vi "Temperature sub final.vi"(8 "error in (no error)":errorcluster, 10 "Numeric 3":i32, 11 "LINX Resource":T1) -> (2 "Numeric 2":i32, 3 "Numeric":dbl)   [LabVIEW 2020]
uses:
  <vilib>/MakerHub/LINX/Private/Type Defs/LINX Ref.ctl
  <vilib>/MakerHub/LINX/Private/Type Defs/Platform.ctl
  <vilib>/MakerHub/LINX/Private/Type Defs/Interface.ctl
  <vilib>/MakerHub/LINX/Private/Device/Type Defs/LINX Device Config.ctl
  <vilib>/MakerHub/LINX/Private/Device/Type Defs/TCP Config.ctl
  <vilib>/MakerHub/LINX/Private/Device/Type Defs/Channels.ctl
  <vilib>/MakerHub/LINX/Public/Peripherals/Analog/Analog Read 1 Chan.vi
  <vilib>/MakerHub/LINX/Public/Peripherals/Analog/Analog Read N Chans.vi
  <vilib>/MakerHub/LINX/Private/Local IO/LinxAnalogRead.vi
  <vilib>/MakerHub/LINX/Public/Utilities/Check Channel.vi
  <vilib>/MakerHub/LINX/Private/Utilties/Generate Error.vi
  <vilib>/MakerHub/LINX/LMH-LINX.lvlib
  <vilib>/MakerHub/LINX/Private/Device/Device.lvlib
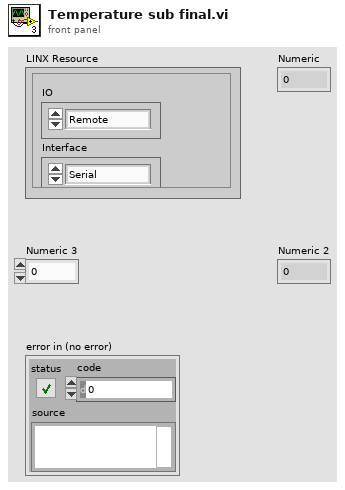
[diagram p1: front panel]
types:
  T1 = typedef "LMH-LINX.lvlib/LINX Ref.ctl" = cluster{"IO":T2, "Interface":T3, "LINX Device Config":T4}
  T2 = typedef "LMH-LINX.lvlib/Platform.ctl" = enum16{"Remote", "Local"}
  T3 = typedef "LMH-LINX.lvlib/Interface.ctl" = enum16{"Serial", "TCP"}
  T4 = typedef "LMH-LINX.lvlib/Device.lvlib/LINX Device Config.ctl" = cluster{"Interface":T3, "COM Port":refnum<visa-resource-name>, "TCP Configuration":T5, "Device Family":u8, "Device ID":u8, "Device Name":string, "TCP Ref":refnum<k5>, "Channels":T6}
  T5 = typedef "LMH-LINX.lvlib/Device.lvlib/TCP Config.ctl" = cluster{"IP Address":string, "Port":u16}
  T6 = typedef "LMH-LINX.lvlib/Channels.ctl" = cluster{"DI":u8[], "DO":u8[], "AI":u8[], "AO":u8[], "PWM":u8[], "QE":u8[], "UART":u8[], "I2C 2":u8[], "SPI":u8[], "CAN":u8[], "Servo":u8[], "AI Ref (V)":dbl, "AI Resolution (Bits)":u8, "AO Ref (V)":dbl, "AO Resolution (Bits)":u8}
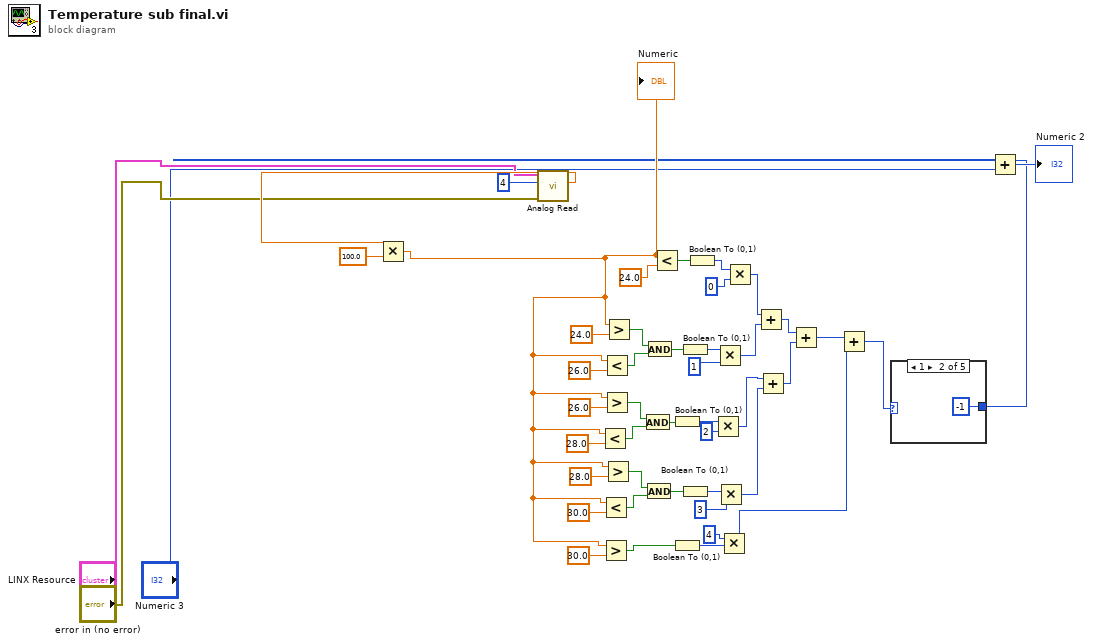
[diagram p0: block diagram]
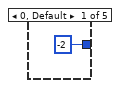
[diagram p2: hidden frame]
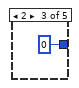
[diagram p3: hidden frame]
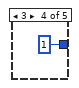
[diagram p4: hidden frame]
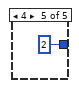
[diagram p5: hidden frame]
diagram:
  n1 = call-poly <vilib>:"Analog Read.vi"("Error In"="error in (no error)", "Analog Channel"=u8 4, "LINX Resource"="LINX Resource") -> ("Voltage"=w47:dbl)  [unwired: 5 in, 3 out]
  n2 = Multiply(x=w47, y=100.0) -> (x*y=w6:dbl)
  "Numeric" <- w6
  n3 = Less?(x=w6, y=28.0) -> (x < y?=w15:bool)
  n4 = Less?(x=w6, y=30.0) -> (x < y?=w19:bool)
  n5 = Greater?(x=w6, y=30.0) -> (0:w23:bool)
  n6 = Less?(x=w6, y=26.0) -> (x < y?=w11:bool)
  n7 = Greater?(x=w6, y=26.0) -> (0:w16:bool)
  n8 = Greater?(x=w6, y=28.0) -> (0:w20:bool)
  n9 = Greater?(x=w6, y=24.0) -> (0:w12:bool)
  n10 = And(x=w16, y=w15) -> (x .and. y?=w25:bool)
  n11 = And(x=w20, y=w19) -> (x .and. y?=w24:bool)
  n12 = And(x=w12, y=w11) -> (x .and. y?=w26:bool)
  n13 = Less?(x=w6, y=24.0) -> (x < y?=w27:bool)
  n14 = Boolean To (0,1)(Boolean=w25) -> (0, 1=w37:i16)
  n15 = Boolean To (0,1)(Boolean=w23) -> (0, 1=w31:i16)
  n16 = Boolean To (0,1)(Boolean=w26) -> (0, 1=w34:i16)
  n17 = Boolean To (0,1)(Boolean=w24) -> (0, 1=w43:i16)
  n18 = Boolean To (0,1)(Boolean=w27) -> (0, 1=w32:i16)
  n19 = Multiply(x=w37, y=i16 2) -> (x*y=w39:i16)
  n20 = Multiply(x=w34, y=i16 1) -> (x*y=w36:i16)
  n21 = Multiply(x=w43, y=i16 3) -> (x*y=w40:i16)
  n22 = Multiply(x=i16 4, y=w31) -> (x*y=w41:i16)
  n23 = Multiply(x=w32, y=i16 0 ("0, 1")) -> (x*y=w33:i16)
  n24 = Add(x=w33, y=w36) -> (x+y=w29:i16)
  n25 = Add(x=w39, y=w40) -> (x+y=w30:i16)
  n26 = Add(x=w29, y=w30) -> (x+y=w28:i16)
  n27 = Add(x=w28, y=w41) -> (x+y=w22:i16)
  n28 = case shown="1" w22 {
    tunnel: [-2 -1 0 1 2] -> w1
    frame 0, Default {
    }
    frame 1 {
    }
    frame 2 {
    }
    frame 3 {
    }
    frame 4 {
    }
  }
  n29 = Add(x=w1, y="Numeric 3") -> (x+y=→"Numeric 2":i32)
